vi "SIM Real LU Factorization.vi"(0 "A":T1) -> (1 "L":T1, 2 "U":T1, 3 "P":i32[][](array[numeric]), 4 "error":i32)   [LabVIEW 2017]
doc: "Performs the LU factorization of <B>A</B>. The data type you wire to the <B>A</B> input determines the polymorphic instance to use."
uses:
  RealMatrix.ctl
  <resource>/lvanlys.dll
  NI_Matrix.lvlib
panel:
  # "LU Factorization"
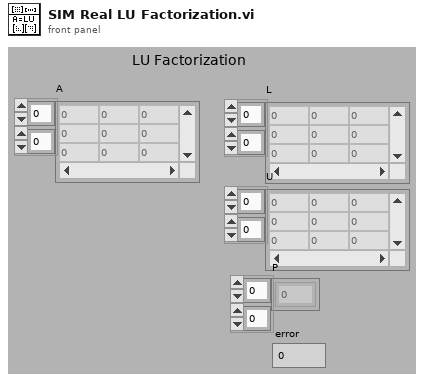
[diagram p1: front panel]
types:
  T1 = typedef "NI_Matrix.lvlib/RealMatrix.ctl" = dbl[][]
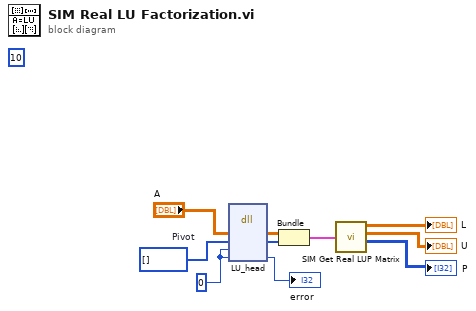
[diagram p0: block diagram]
diagram:
  w9 = 0 ("error")
  w10 = i32[] []  # Pivot
  (unwired) 10
  n1 = dll-call lib="C:/Program Files (x86)/National Instruments/LabVIEW 2017/resource/lvanlys.*" fn="LU_head"("output param"="A", "Pivot"=w10, "sign"=w9, "error"=w9) -> ("output param"=w7:T1, "Pivot"=w6:i32[], "error"=→"error":i32)  [unwired: 5 in, 2 out]
  n2 = Bundle("output param"=w7, "Pivot"=w6) -> (w4:cluster{"output param":T1, "Pivot":i32[]})  [unwired: 1 in]
  n3 = call "SIM Get Real LUP Matrix.vi"("LU Info"=w4) -> ("L"=→"L":T1, "U"=→"U":T1, "P"=→"P":i32[][])  [unwired: 1 in]
